vi "Face_Colors.vi"(9 "offset":dbl=50.0, 11 "Z Value":dbl) -> (0 "right":u32, 1 "top":u32, 2 "left":u32, 3 "bottom":u32)   [LabVIEW 2022 SP3]
uses:
  Perspective_Globals.vi
panel:
  out "Array":u32[](array[colorbox])
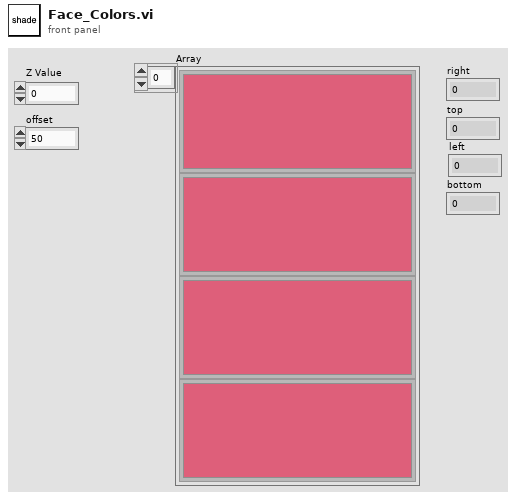
[diagram p1: front panel]
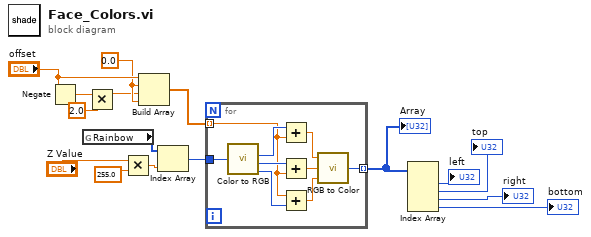
[diagram p0: block diagram]
diagram:
  w13 = 0.0 ("element")
  n1 = Negate(x="offset") -> (-x=w15:dbl)
  n2 = global read "Perspective_Globals.vi" "Rainbow"() -> (w6:u32[])
  n3 = Multiply(x=w15, y=2.0) -> (x*y=w12:dbl)
  n4 = Multiply(x="Z Value", y=255.0) -> (x*y=w7:dbl)
  n5 = Build Array("offset", w13, w12, w13) -> (w16:dbl[])
  n6 = Index Array(array=w6, index=w7) -> (element=w5:u32)
  n7 = for {
    tunnel: w5 -> [w21]
    tunnel: w16 -> [w17] mode=indexing
    tunnel: [w20] -> w10 mode=indexing
    n8 = call <vilib>:"Color to RGB.vi"("Color"=w21) -> ("R"=w22:u8, "G"=w19:u8, "B"=w24:u8)  [unwired: 1 out]
    n9 = Add(x=w22, y=w17) -> (x+y=w23:dbl)
    n10 = Add(x=w19, y=w17) -> (x+y=w18:dbl)
    n11 = Add(x=w17, y=w24) -> (x+y=w25:dbl)
    n12 = call <vilib>:"RGB to Color.vi"("B"=w25, "G"=w18, "R"=w23) -> ("Color"=w20:u32)
  }
  "Array" <- w10
  n13 = Index Array(array=w10) -> (element #1=→"left":u32, element #2=→"top":u32, element #3=→"right":u32, element #4=→"bottom":u32)  [unwired: 4 in]
